vi "writeU16FIFO.vi"(8 "error in (no error)":errorcluster, 9 "Timeout":i32, 10 "Data":u16[](array[numeric]), 11 "ModbusSubnetDTxDataFIFO in":refnum<class "ModbusSubnetDTxDataFIFO.lvclass">) -> (0 "error out":errorcluster, 2 "ElementsRemaining":u32, 3 "ModbusSubnetDTxDataFIFO out":refnum<class "ModbusSubnetDTxDataFIFO.lvclass">)   [LabVIEW 2016, in "ModbusSubnetDTxDataFIFO.lvclass"]
uses:
  ModbusSubnetDTxDataFIFO.lvclass
  FPGA/FPGA.lvclass
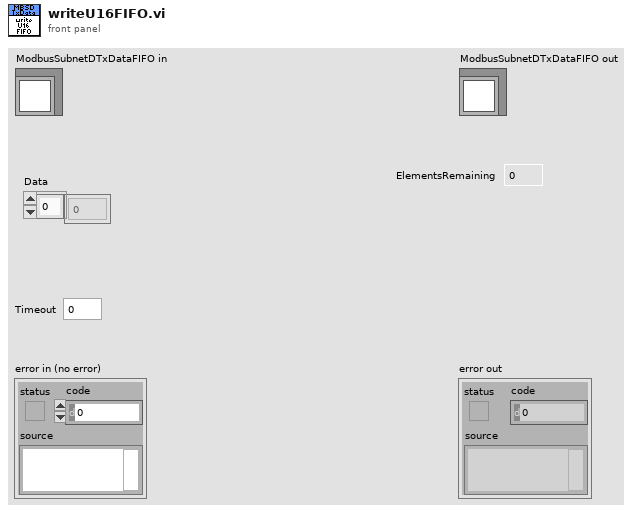
[diagram p1: front panel]
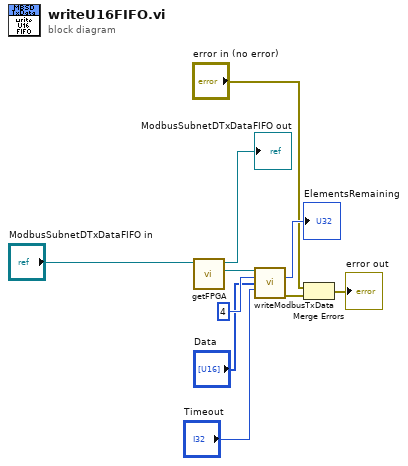
[diagram p0: block diagram]
diagram:
  n1 = call "getFPGA.vi"("ModbusSubnetDTxDataFIFO in"="ModbusSubnetDTxDataFIFO in") -> ("FPGA"=w9:refnum<class "FPGA.lvclass">, "ModbusSubnetDTxDataFIFO out"=→"ModbusSubnetDTxDataFIFO out":refnum<class "ModbusSubnetDTxDataFIFO.lvclass">)  [unwired: 9 in]
  n2 = call "writeModbusTxData.vi"("FPGA in"=w9, 5:u16 4 ("Subnet"), 7:"Data", "Timeout (ms)"="Timeout") -> ("Empty Elements Remaining"=→"ElementsRemaining":u32, "error out"=w3:errorcluster)  [unwired: 9 in, 1 out]
  n3 = Merge Errors("error in (no error)", w3) -> (→"error out":errorcluster)
